vi "Filter Items.vi"(11 "Item Graph In":T1[](array[typedef])) -> (3 "Item Graph":T1[](array[typedef]))   [LabVIEW 2020, in "TypeGraph.lvlib"]
uses:
  TypeGraph.lvlib
  Type Reflection Item.ctl
  <vilib>/Utility/Data Type/NI_Data Type.lvlib
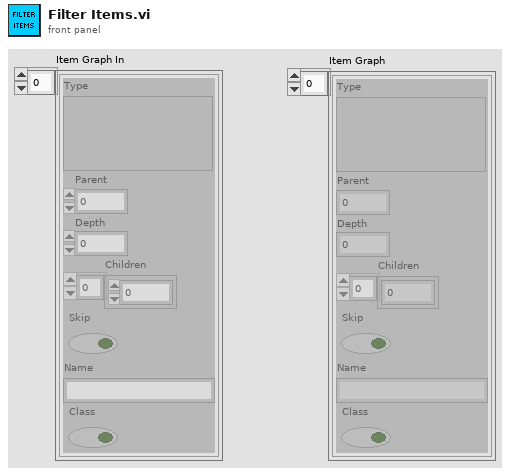
[diagram p1: front panel]
types:
  T1 = typedef "TypeGraph.lvlib/Type Reflection Item.ctl" = cluster{"Type":variant, "Parent":i32, "Depth":i32, "Children":i32[], "Skip":bool, "Name":string, "Class":bool}
  T2 = typedef "NI_Data Type.lvlib/Data Type.ctl" = enum8{"Invalid Type", "Void", "I8", "I16", "I32", "I64", "U8", "U16", "U32", "U64", "Single Float", "Double Float", "Extended Float", "Single Complex", "Double Complex", "Extended Complex", "Enum U8", "Enum U16", "Enum U32", "Enum U64", "Single Float With Unit", "Double Float With Unit", "Extended Float With Unit", "Single Complex with Unit", "Double Complex with Unit", "Extended Complex with Unit", "Boolean", "String", "Path", "Picture", "Tag", "Array", "Cluster", "Variant", "LV Variant", "Waveform", "Timestamp", "Digital Waveform", "Digital Data", "ExpressData", "Refnum", "External Data", "VI", "Poly VI", "LabVIEW Class Instance", "Fixed Point", "Set Collection", "Map Collection"}
  T3 = typedef "NI_Data Type.lvlib/Refnum Type.ctl" = enum16{"NotARefnum", "UnknownRefnum", "Generic", "Datalog", "ByteStream", "Device", "Occurence", "TCPNetConnection", "Auto", "Menu", "Imaq", "Hardware", "DataSocket", "Visa", "IVI", "UDPNetConnection", "Notifier", "Queue", "Irda", "EventReg", "DotNet", "UserEvent", "Callback", "UNUSED_EMPTY_POSITION", "BlueToothNetConnection", "LVObjApp", "LVObjVI", "LVObjUnknown", "GenericClass", "UserDefinedRefnumTag", "DataValue", "RT FIFO", "TDMS File", "PythonSessionRefnum"}
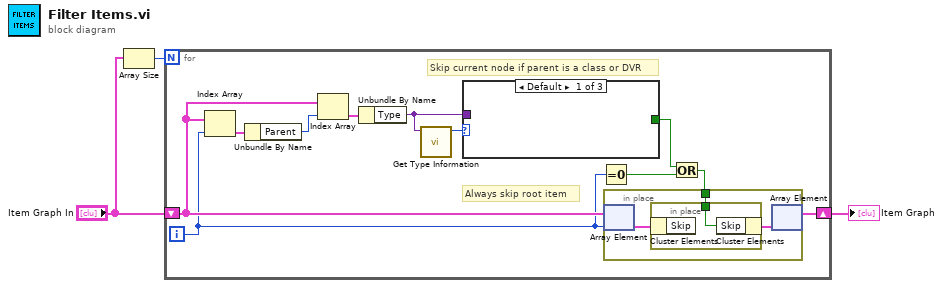
[diagram p0: block diagram]
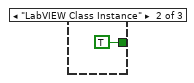
[diagram p2: hidden frame]
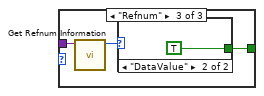
[diagram p3: hidden frame]
diagram:
  n1 = Array Size(array="Item Graph In") -> (size(s)=w3:i32)
  n2 = for {
    N: w3 -> [_]
    shift-right: [w8] -> w2
    shift-left: "Item Graph In" -> [w9]
    i -> [w7]
    # "Always skip root item"
    # "Skip current node if parent is a class or DVR"
    n3 = Index Array(array=w9, index=w7) -> (element=w14:T1)
    n4 = Unbundle By Name(w14) -> ("Parent"=w13:i32)
    n5 = Index Array(array=w9, index=w13) -> (element=w12:T1)
    n6 = Unbundle By Name(w12) -> ("Type"=w10:variant)
    n7 = call <vilib>:"Get Type Information.vi"("variant"=w10) -> ("type"=w11:T2)  [unwired: 6 in, 4 out]
    n8 = case shown="Default" w11 {
      tunnel: w10 -> [_ _ w22]
      tunnel: [_ TRUE w20] -> w5
      frame Default {
      }
      frame "LabVIEW Class Instance" {
      }
      frame "Refnum" {
        n9 = call <vilib>:"Get Refnum Information.vi"("variant"=w22) -> ("reference type"=w21:T3)  [unwired: 7 in, 3 out]
        n10 = case shown="\"DataValue\"" w21 {
          tunnel: [_ TRUE] -> w20
          frame Default {
          }
          frame "DataValue" {
          }
        }
      }
    }
    n11 = Equal To 0?(x=w7) -> (x = 0?=w4:bool)
    n12 = Or(x=w5, y=w4) -> (x .or. y?=w6:bool)
    n13 = in-place {
      in-place-border: w6 -> [w15]
      n14 = in-place-array #1(w9, w7) -> (w17:T1)
      n15 = in-place {
        in-place-border: w15 -> [w18]
        n16 = in-place-cluster #2(w17) -> ()  [unwired: 1 out]
        n17 = in-place-cluster #2("Skip"=w18) -> (w16:T1)
      }
      n18 = in-place-array #1(w16) -> (w8:T1[])  [unwired: 1 out]
    }
  }
  "Item Graph" <- w2
